vi "UpdateActualDepsList.vi"(6 "StatusIndicator Ref":refnum<vi>, 8 "error in (no error)":errorcluster, 10 "LibraryNames":string[](array[string]), 11 "Workspace Path":path=path "E:/sw-deps-monitor") -> (0 "error out":errorcluster)   [LabVIEW 2023, in "Reusables.lvlib"]
uses:
  Reusables/Reusables.lvlib
  <vilib>/Utility/config.llb/NI_LVConfig.lvlib
  CheckModifiedVIs/CheckModifiedVIs.lvlib
panel:
  out "Status Indicator":string
  # "Leave Empty to update all Libraries"
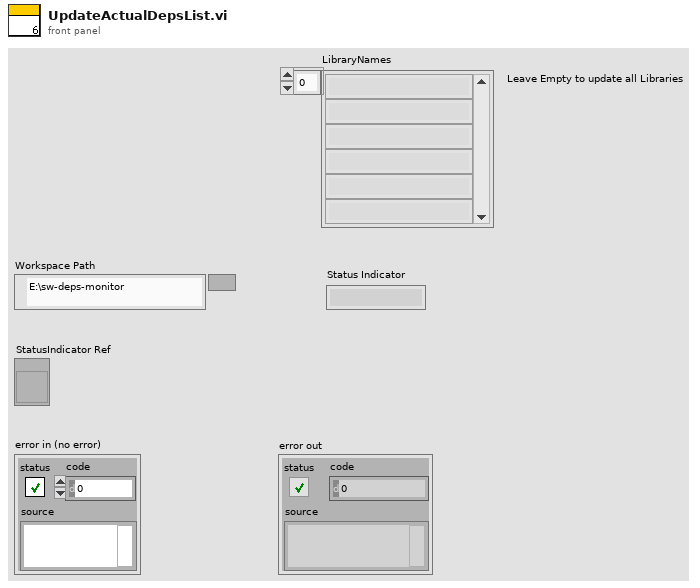
[diagram p1: front panel]
types:
  T1 = typedef "NI_LVConfig.lvlib/Config Data RefNum.ctl" = refnum<k1>
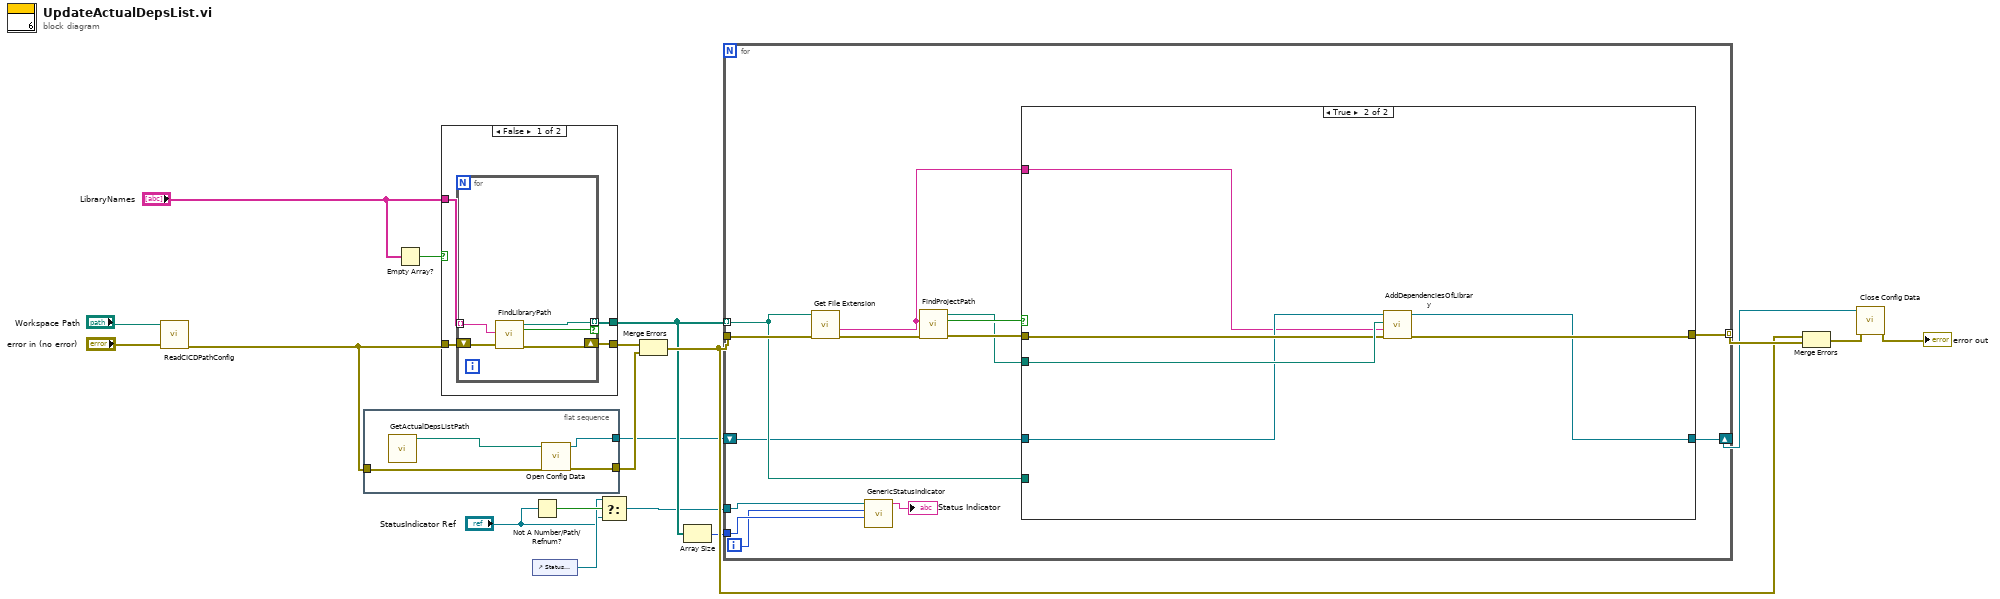
[diagram p0: block diagram]
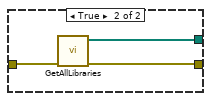
[diagram p2: hidden frame]
diagram:
  n1 = call "ReadCICDPathConfig.vi"("error in (no error)"="error in (no error)", "Workspace Path"="Workspace Path") -> ("error out"=w3:errorcluster)  [unwired: 8 in, 1 out]
  n2 = flat-sequence {
    tunnel: [w23] -> w1
    tunnel: [w22] -> w2
    tunnel: w3 -> [w20]
    frame #0 {
      n3 = call "GetActualDepsListPath.vi"() -> ("Path"=w21:path)  [unwired: 11 in]
      n4 = call <vilib>:"Open Config Data.vi"("error in (no error)"=w20, "configuration file path"=w21) -> ("error out"=w22:errorcluster, "refnum"=w23:T1)  [unwired: 7 in, 1 out]
    }
  }
  n5 = Empty Array?(array="LibraryNames") -> (empty?=w14:bool)
  n6 = case shown="False" w14 {
    tunnel: w3 -> [w27 w35]
    tunnel: [w25 w34] -> w11
    tunnel: "LibraryNames" -> [w26 _]
    tunnel: [w24 w33] -> w12
    frame False {
      n7 = for {
        tunnel: w26 -> [w31] mode=indexing
        shift-right: [w30] -> w24
        shift-left: w27 -> [w32]
        tunnel: [w29] -> w25 mode=indexing if=w28
        n8 = call "FindLibraryPath.vi"("error in (no error)"=w32, "Library Name"=w31) -> ("error out"=w30:errorcluster, "Found?"=w28:bool, "Library Path"=w29:path)  [unwired: 7 in]
      }
    }
    frame True {
      n9 = call "GetAllLibraries.vi"("error in (no error)"=w35) -> ("error out"=w33:errorcluster, "Lvlib paths"=w34:path[])  [unwired: 9 in]
    }
  }
  n10 = Not A Number/Path/Refnum?(number/path/refnum="StatusIndicator Ref") -> (NaN/Path/Refnum?=w9:bool)
  n11 = control-ref of="Status Indicator"() -> (w8:refnum<vi>)
  n12 = Select(t=w8, s=w9, f="StatusIndicator Ref") -> (s? t:f=w6:refnum<vi>)
  n13 = Merge Errors(w12, w2) -> (w15:errorcluster)
  n14 = Array Size(array=w11) -> (size(s)=w10:i32)
  n15 = for {
    tunnel: w15 -> [w49]
    tunnel: w11 -> [w47] mode=indexing
    tunnel: [w48] -> w19 mode=indexing
    shift-right: [w41] -> w16
    shift-left: w1 -> [w42]
    tunnel: w6 -> [w39]
    tunnel: w10 -> [w38]
    i -> [w37]
    n16 = call <vilib>:"Get File Extension.vi"("error in (no error)"=w49, "file"=w47) -> ("error out"=w46:errorcluster, "filename without extension"=w40:string)  [unwired: 5 in, 3 out]
    n17 = call "GenericStatusIndicator.vi"("Total"=w38, "Current Iteration"=w37, "String in"=w39) -> ("Status"=→"Status Indicator":string)  [unwired: 8 in]
    n18 = call "FindProjectPath.vi"("error in (no error)"=w46, "Library Name"=w40) -> ("error out"=w44:errorcluster, "Found?"=w45:bool, "Project Path"=w43:path)  [unwired: 7 in]
    n19 = case shown="True" w45 {
      tunnel: w44 -> [w51 w56]
      tunnel: w47 -> [_ _]
      tunnel: [w51 w55] -> w48
      tunnel: w43 -> [_ w57]
      tunnel: w42 -> [w50 w54]
      tunnel: [w50 w53] -> w41
      tunnel: w40 -> [_ w52]
      frame False {
      }
      frame True {
        n20 = call "AddDependenciesOfLibrary.vi"("error in (no error)"=w56, "LibraryName"=w52, "Project Path"=w57, "Config Refnum in"=w54) -> ("error out"=w55:errorcluster, "Config Refnum out"=w53:T1)  [unwired: 5 in, 1 out]
      }
    }
  }
  n21 = Merge Errors(w15, w19) -> (w18:errorcluster)
  n22 = call <vilib>:"Close Config Data.vi"("error in (no error)"=w18, "refnum"=w16) -> ("error out"=→"error out":errorcluster)  [unwired: 8 in, 1 out]
